vi "remove broken property items.vi"(8 "error in (no error)":errorcluster, 11 "VI in":refnum<vi>) -> (0 "error out":errorcluster, 3 "VI out":refnum<vi>)   [LabVIEW 2013, in "NISE Tools Scripting.lvlib"]
uses:
  NISE Tools Scripting.lvlib
  <vilib>/Utility/traverseref.llb/TRef TravTarget.ctl
  <vilib>/Utility/traverseref.llb/VI Scripting - Traverse.lvlib
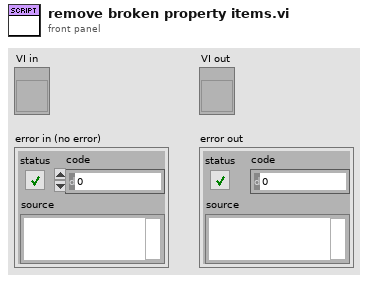
[diagram p1: front panel]
types:
  T1 = typedef "TRef TravTarget.ctl" = enum16{"FP", "BD", "Other"}
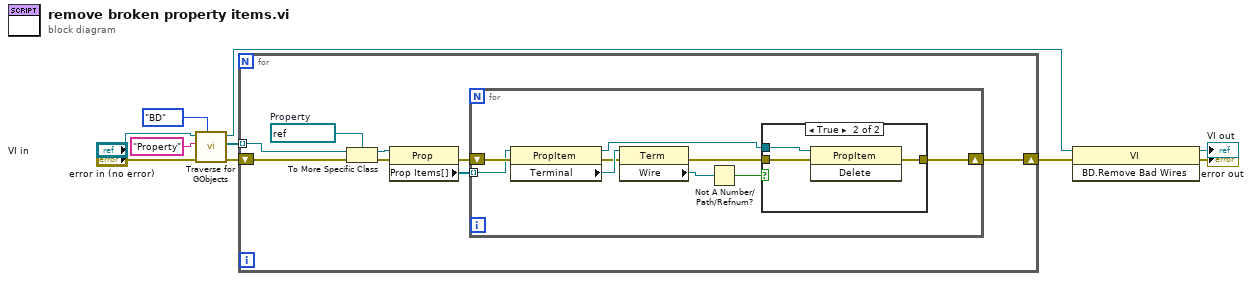
[diagram p0: block diagram]
diagram:
  n1 = call <vilib>:"Traverse for GObjects.vi"("Traverse Target"=TRef_TravTarget."BD", "error in (no error)"="error in (no error)", "Class Name"="Property", "VI Refnum"="VI in") -> ("error out"=w2:errorcluster, "References"=w4:refnum<vi>[], "dup VI Refnum"=w6:refnum<vi>)  [unwired: 4 in, 1 out]
  n2 = for {
    shift-right: [w11] -> w3
    shift-left: w2 -> [w18]
    tunnel: w4 -> [w17] mode=indexing
    w16 = refnum<vi> refnum  # Property
    n3 = To More Specific Class(target class=w16, reference=w17, error in=w18) -> (specific class reference=w15:refnum<vi>, error out=w14:errorcluster)
    n4 = property class="Prop"(reference=w15, error in=w14) -> (error out=w13:errorcluster, "Prop Items[]"=w12:refnum<vi>[])  [unwired: 1 out]
    n5 = for {
      shift-right: [w19] -> w11
      shift-left: w13 -> [w27]
      tunnel: w12 -> [w26] mode=indexing
      n6 = property class="PropItem"(reference=w26, error in=w27) -> (reference out=w20:refnum<vi>, error out=w23:errorcluster, "Terminal"=w25:refnum<vi>)
      n7 = property class="Term"(reference=w25, error in=w23) -> (error out=w21:errorcluster, "Wire"=w24:refnum<vi>)  [unwired: 1 out]
      n8 = Not A Number/Path/Refnum?(number/path/refnum=w24) -> (NaN/Path/Refnum?=w22:bool)
      n9 = case shown="True" w22 {
        tunnel: w21 -> [w28 w31]
        tunnel: w20 -> [_ w30]
        tunnel: [w28 w29] -> w19
        frame False {
        }
        frame True {
          n10 = invoke class="PropItem" method="Delete"(reference=w30, error in=w31) -> (error out=w29:errorcluster)  [unwired: 1 in, 2 out]
        }
      }
    }
  }
  n11 = invoke class="VI" method="BD.Remove Bad Wires"(reference=w6, error in=w3) -> (reference out=→"VI out":refnum<vi>, error out=→"error out":errorcluster)  [unwired: 1 in, 1 out]
